vi "Configure Measurement.vi"(8 "error in (no error)":errorcluster, 10 "Window Handle":i32, 11 "Config File Path":path=path "TestStand.ini") -> (0 "error out":errorcluster, 1 "Show UI?":bool, 2 "Device Names":string[](array[string]), 3 "Measurement Name":string)   [LabVIEW 2016, in "Measurement Setup Controller.lvlib" / "Measurement Setup.lvclass"]
uses:
  Measurement Setup.lvclass
  MAL-Framework/user.lib/Common Components/Msmt Configuration/Controller Configuration.lvclass
  C:/Program Files (x86)/National Instruments/LabVIEW 2016/user.lib/Configuration Dialog Actor/Configuration.lvclass
  UI/Measurement Setup UI.lvclass
  \\Mac\Home/Documents/MAL-Framework/user.lib/Common Components/User Interface/UI.lvclass
  <vilib>/ActorFramework/LastAck/Last Ack.lvclass
  \\Mac\Home/Documents/MAL-Framework/user.lib/Common Components/Controller/Controller.lvclass
  C:/Program Files (x86)/National Instruments/LabVIEW 2016/vi.lib/ActorFramework/Actor/Actor.lvclass
  <vilib>/ActorFramework/Message Queue/Message Queue.lvclass/Message Queue.ctl
  UI/Measurement Setup UI.lvclass/Measurement Setup UI.ctl
  <vilib>/ActorFramework/Message Dequeuer/Message Dequeuer.lvclass/Message Dequeuer.ctl
  <vilib>/ActorFramework/LastAck/Last Ack.lvclass/Last Ack.ctl
  Measurement Setup.lvclass/Measurement Setup.ctl
  Measurement Data/Measurement Data.lvclass/Measurement Data.ctl
  <vilib>/ActorFramework/Message Priority Queue/Priority Dequeue.vi
  Measurement Data/Measurement Data.lvclass
  <vilib>/ActorFramework/Message Queue/Message Queue.lvclass
  <vilib>/ActorFramework/Message Dequeuer/Message Dequeuer.lvclass
  <vilib>/ActorFramework/Actor/Actor.lvclass
  MAL-Framework/user.lib/Common Components/Controller/Controller.lvclass
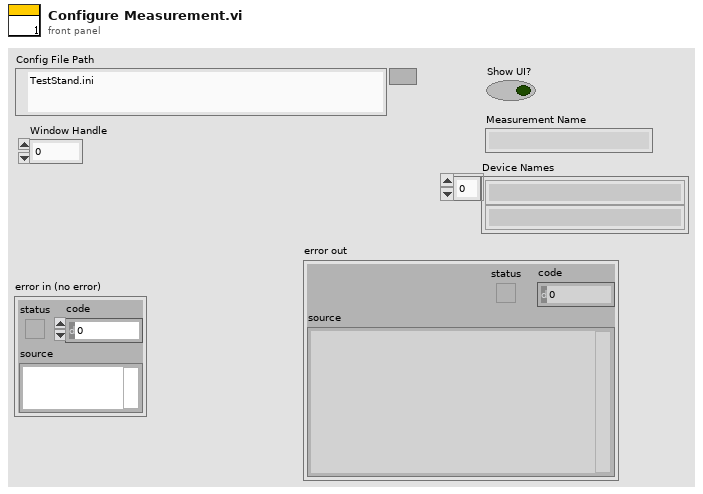
[diagram p1: front panel]
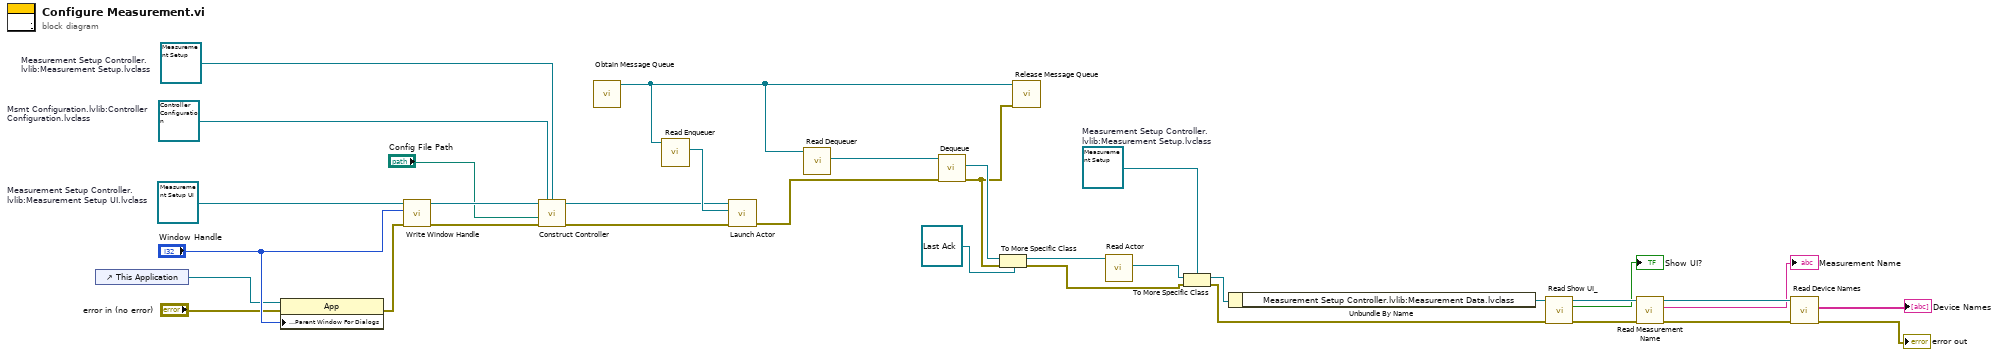
[diagram p0: block diagram]
diagram:
  w27 = refnum<class "Measurement Setup.lvclass"> refnum  # Measurement Setup Controller.lvlib:Measurement Setup.lvclass
  w34 = refnum<class "Measurement Setup UI.lvclass"> refnum  # Measurement Setup Controller.lvlib:Measurement Setup UI.lvclass
  w7 = refnum<class "Measurement Setup.lvclass"> refnum  # Measurement Setup Controller.lvlib:Measurement Setup.lvclass
  w6 = refnum<class "Controller Configuration.lvclass"> refnum  # Msmt Configuration.lvlib:Controller Configuration.lvclass
  n1 = control-ref of="This Application"() -> (w12:refnum<vi>)
  n2 = property class="App"(reference=w12, error in="error in (no error)", "Application:Parent Window For Dialogs"="Window Handle") -> (error out=w11:errorcluster)  [unwired: 1 out]
  n3 = call "Write Window Handle.vi"("error in (no error)"=w11, "Window Handle"="Window Handle", "Measurement Setup UI in"=w34) -> ("error out"=w4:errorcluster, "Measurement Setup UI out"=w8:refnum<class "Measurement Setup UI.lvclass">)  [unwired: 7 in]
  n4 = call "Construct Controller.vi"("UI.lvclass"=w8, "error in (no error)"=w4, "Root Path"="Config File Path", "Configuration.lvlib:Configuration.lvclass"=w6, "Controller Actor.lvlib:Controller.lvclass"=w7) -> ("error out"=w2:errorcluster, "Controller Actor.lvlib:Controller.lvclass 2"=w1:refnum<class "Measurement Setup.lvclass">)  [unwired: 4 in, 1 out]
  n5 = call <vilib>:"Obtain Message Queue.vi"() -> ("Message Queue"=w33:refnum<class "Message Queue.lvclass">)  [unwired: 10 in, 1 out]
  n6 = call <vilib>:"Read Enqueuer.vi"("Message Queue"=w33) -> ("Message Enqueuer"=w10:refnum<class "Message Enqueuer.lvclass">)  [unwired: 10 in]
  n7 = call <vilib>:"Launch Actor.vi"("error in (no error)"=w2, "Actor-to-Caller Enqueuer"=w10, "Actor"=w1) -> ("error out"=w9:errorcluster)  [unwired: 7 in, 1 out]
  n8 = call <vilib>:"Read Dequeuer.vi"("Message Queue"=w33) -> ("Message Dequeuer"=w32:refnum<class "Message Dequeuer.lvclass">)  [unwired: 10 in]
  n9 = call <vilib>:"Dequeue.vi"("error in (no error)"=w9, "Message Dequeuer in"=w32) -> ("error out"=w15:errorcluster, "Message"=w31:refnum<class "Message.lvclass">)  [unwired: 5 in, 3 out]
  n10 = To More Specific Class(target class=refnum<class "Last Ack.lvclass"> refnum ("Last Ack"), reference=w31, error in=w15) -> (specific class reference=w29:refnum<class "Last Ack.lvclass">, error out=w19:errorcluster)
  n11 = call <vilib>:"Release Message Queue.vi"("error in (no error)"=w15, "Message Queue"=w33) -> ()  [unwired: 8 in, 2 out]
  n12 = call <vilib>:"Read Actor.vi"("Last Ack"=w29) -> ("Actor"=w28:refnum<class "Actor.lvclass">)  [unwired: 10 in]
  n13 = To More Specific Class(target class=w27, reference=w28, error in=w19) -> (specific class reference=w26:refnum<class "Measurement Setup.lvclass">, error out=w22:errorcluster)
  n14 = Unbundle By Name(w26) -> ("Measurement Setup Controller.lvlib:Measurement Data.lvclass"=w25:refnum<class "Measurement Data.lvclass">)
  n15 = call "Read Show UI_.vi"("error in (no error)"=w22, "Measurement Data in"=w25) -> ("error out"=w21:errorcluster, "Show UI?"=→"Show UI?":bool, "Measurement Data out"=w24:refnum<class "Measurement Data.lvclass">)  [unwired: 7 in]
  n16 = call "Read Measurement Name.vi"("error in (no error)"=w21, "Measurement Data in"=w24) -> ("error out"=w20:errorcluster, "Measurement Name"=→"Measurement Name":string, "Measurement Data out"=w23:refnum<class "Measurement Data.lvclass">)  [unwired: 7 in]
  n17 = call "Read Device Names.vi"("error in (no error)"=w20, "Measurement Data in"=w23) -> ("error out"=→"error out":errorcluster, "Device Names"=→"Device Names":string[])  [unwired: 7 in, 1 out]
